vi "Get Offset Past Last Channel.vi"(8 "error in (no error)":errorcluster, 11 "Transfer Configuration in":refnum<class "Configuration.Transfer.lvclass">) -> (0 "error out":errorcluster, 2 "last offset":u64, 3 "Transfer Configuration out":refnum<class "Configuration.Transfer.lvclass">)   [LabVIEW 2016, in "Configuration.Transfer.lvclass"]
uses:
  Configuration.Transfer.lvclass
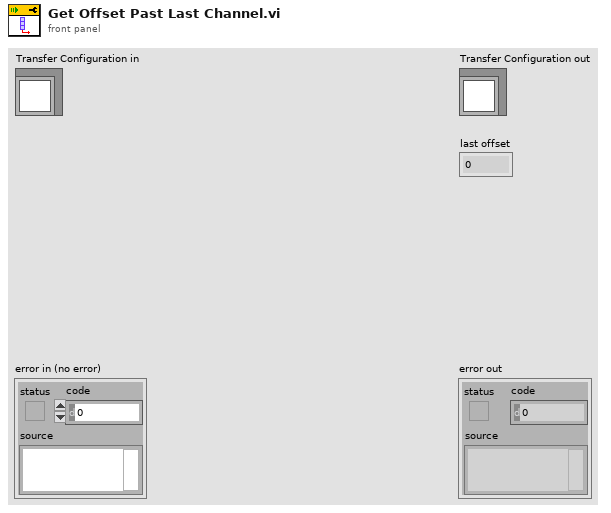
[diagram p1: front panel]
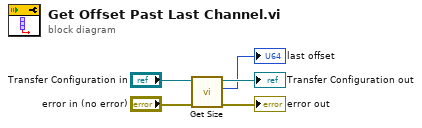
[diagram p0: block diagram]
diagram:
  n1 = call "Get Size.vi"("error in (no error)"="error in (no error)", "Transfer Configuration in"="Transfer Configuration in") -> ("error out"=→"error out":errorcluster, "size in bytes"=→"last offset":u64, "Transfer Configuration out"=→"Transfer Configuration out":refnum<class "Configuration.Transfer.lvclass">)  [unwired: 7 in]
